vi "Read Single Item.vi"(8 "error in (no error)":errorcluster, 11 "Tree in":refnum<class "Tree.lvclass">) -> (0 "error out":errorcluster, 2 "TreeItem":T1, 3 "Tree out":refnum<class "Tree.lvclass">)   [LabVIEW 2024, in "Tree.lvclass"]
uses:
  Tree.lvclass
  Type Def/Tree Item.ctl
  Tree.lvclass/Tree.ctl
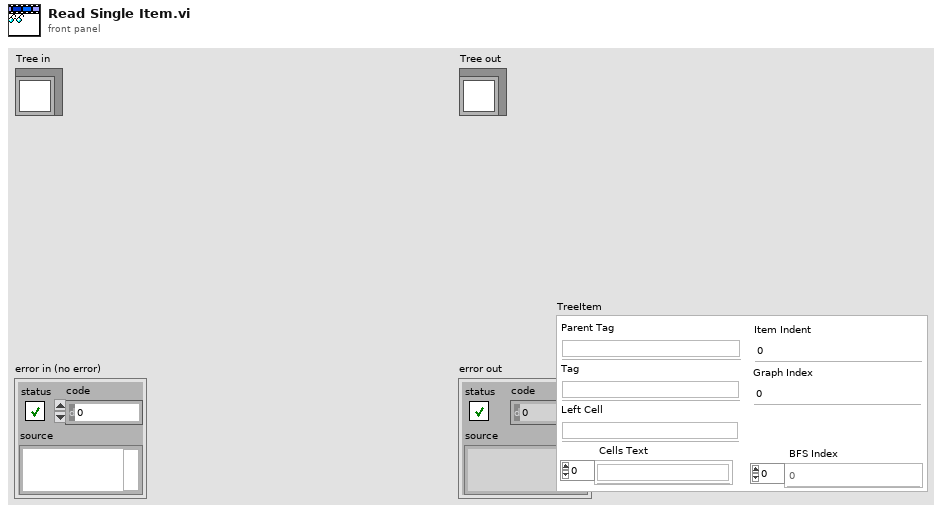
[diagram p1: front panel]
types:
  T1 = typedef "Tree Item.ctl" = cluster{"Parent Tag":string, "Tag":string, "Left Cell":string, "Cells Text":string[], "BFS Index":i32[], "Graph Index":i32, "Item Indent":i32}
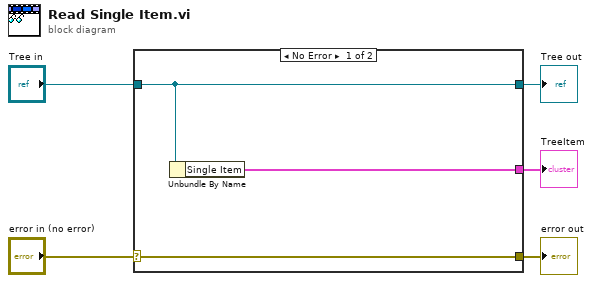
[diagram p0: block diagram]
diagram:
  n1 = case shown="No Error" "error in (no error)" {
    selector: "error in (no error)" -> [w8 w9]
    tunnel: [w8 w9] -> w4
    tunnel: [w7 w10] -> w2
    tunnel: "Tree in" -> [w7 w10]
    tunnel: [w6 _] -> w1
    frame No Error {
      n2 = Unbundle By Name(w7) -> ("Single Item"=w6:T1)
    }
    frame Error {
    }
  }
  "error out" <- w4
  "Tree out" <- w2
  "TreeItem" <- w1
